vi "Busy.vi"(8 "error in (no error)":errorcluster, 11 "Camera_Prime95B in":refnum<class "Camera_Prime95B.lvclass">) -> (0 "error out":errorcluster, 2 "isBusy?":bool, 3 "Camera_Prime95B out":refnum<class "Camera_Prime95B.lvclass">)   [LabVIEW 2020, in "Camera_Prime95B.lvlib" / "Camera_Prime95B.lvclass"]
uses:
  Camera_Prime95B.lvclass
  E:/Development/DevHardSoftware/MMicroscopyAF/Model/Real Hardware/Camera_Prime95B/Camera_Prime95B/Dependencies/PVCamNET.dll
  Dependencies/PVCamNET.dll
  HAL Layer/Component/Camera/Camera/Camera.lvclass
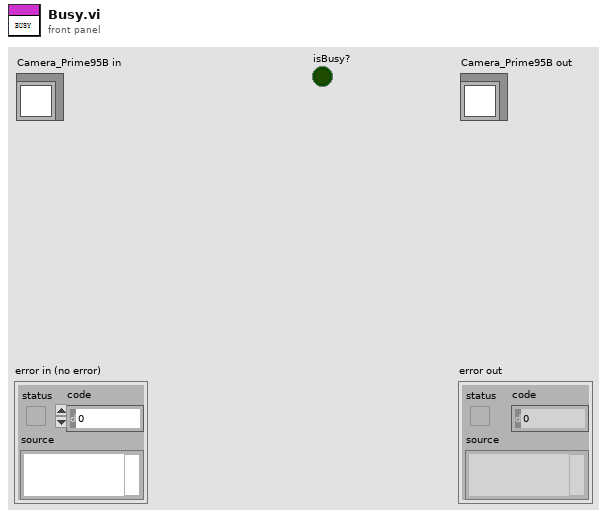
[diagram p1: front panel]
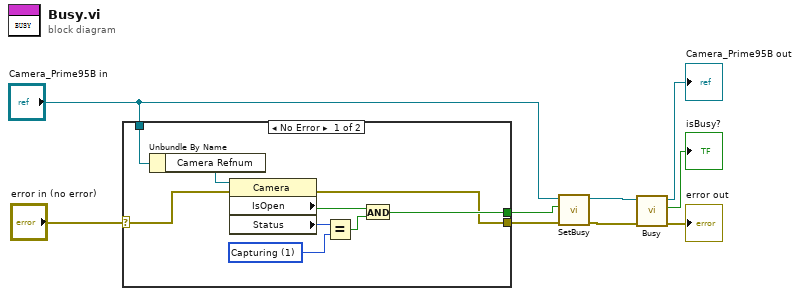
[diagram p0: block diagram]
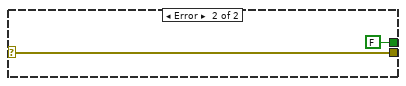
[diagram p2: hidden frame]
diagram:
  n1 = case shown="No Error" "error in (no error)" {
    selector: "error in (no error)" -> [w10 w20]
    tunnel: [w11 w20] -> w3
    tunnel: "Camera_Prime95B in" -> [w18 _]
    tunnel: [w12 FALSE] -> w1
    frame No Error {
      w14 = 1 items=["Idle", "Capturing"] ("Status")
      n2 = Unbundle By Name(w18) -> ("Camera Refnum"=w13:refnum<k24>)
      n3 = property class="Camera"(reference=w13, error in=w10) -> (error out=w11:errorcluster, "IsOpen"=w16:bool, "Status"=w15:i32)  [unwired: 1 out]
      n4 = Equal?(x=w15, y=w14) -> (x = y?=w17:bool)
      n5 = And(x=w16, y=w17) -> (x .and. y?=w12:bool)
    }
    frame Error {
    }
  }
  n6 = call-dynamic "SetBusy.vi"("error in (no error)"=w3, "isBusy?"=w1, "Device in"="Camera_Prime95B in") -> ("error out"=w2:errorcluster, "Device out"=w4:refnum<class "Camera_Prime95B.lvclass">)  [unwired: 7 in]
  n7 = call-parent "Busy.vi"("error in (no error)"=w2, "Device in"=w4) -> ("error out"=→"error out":errorcluster, "isBusy?"=→"isBusy?":bool, "Device out"=→"Camera_Prime95B out":refnum<class "Camera_Prime95B.lvclass">)  [unwired: 7 in]
